vi "Initialise Spectrum Notifier).vi"(8 "error in (no error)":errorcluster) -> (0 "error out":errorcluster)   [LabVIEW 2016]
uses:
  Application Control/Application Globals.vi
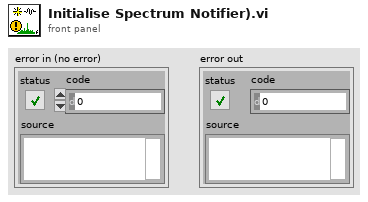
[diagram p1: front panel]
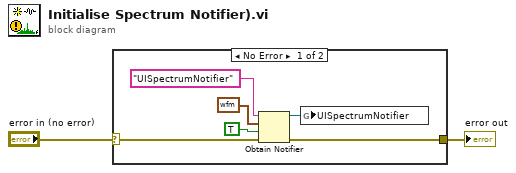
[diagram p0: block diagram]
diagram:
  n1 = case shown="No Error" "error in (no error)" {
    selector: "error in (no error)" -> [w3 w9]
    tunnel: [w8 w9] -> w1
    frame No Error {
      n2 = Obtain Notifier(name (unnamed)="UISpectrumNotifier", notification data type=waveform(dbl) {"t0"=timestamp(0 s since 1904-01-01), "dt"=1.0, "Y"=[]} ("data out"), create if not found? (T)=TRUE, error in (no error)=w3) -> (notifier out=w5:refnum<notifier>, error out=w8:errorcluster)  [unwired: 1 out]
      n3 = global write "Application Globals.vi" "UISpectrumNotifier"(w5) -> ()
    }
    frame Error {
    }
  }
  "error out" <- w1
